vi "Contour Line_Find Intersected Edges.vi"(8 "height in":dbl, 9 "Z":dbl[][](array[numeric]), 10 "Y":dbl[][](array[numeric]), 11 "X":dbl[][](array[numeric])) -> (0 "height out":dbl, 2 "Intersected Edges":T1(array[cluster]), 3 "Contour Points":cluster{"x":dbl, "y":dbl}[](array[cluster]))   [LabVIEW 2020, in "NI_AAL_Geometry.lvlib"]
uses:
  <vilib>/Analysis/NI_AAL_Geometry.lvlib
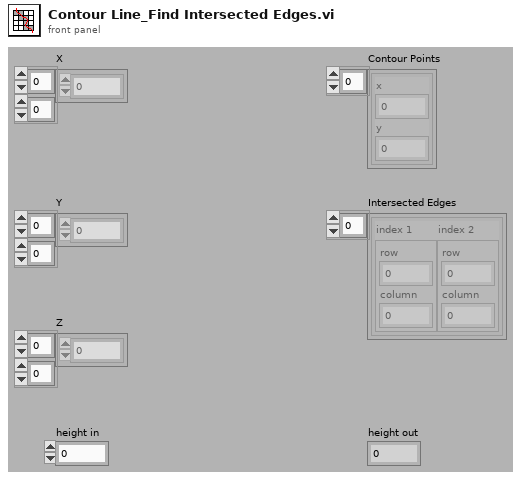
[diagram p1: front panel]
types:
  T1 = cluster{"index 1":cluster{"row":i32, "column":i32}, "index 2":cluster{"row":i32, "column":i32}}[]
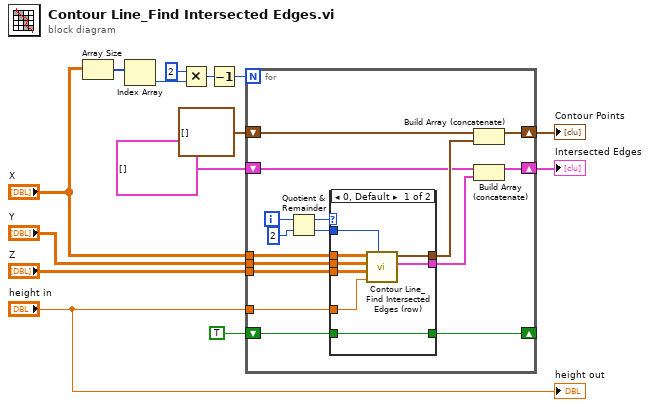
[diagram p0: block diagram]
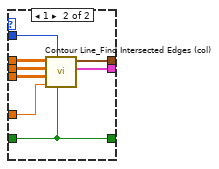
[diagram p2: hidden frame]
diagram:
  n1 = Array Size(array="X") -> (size(s)=w14:i32[])
  n2 = Index Array(array=w14) -> (element=w13:i32)  [unwired: 1 in]
  n3 = Multiply(x=2, y=w13) -> (x*y=w11:i32)
  n4 = Decrement(x=w11) -> (x-1=w10:i32)
  n5 = for {
    N: w10 -> [_]
    tunnel: "X" -> [w26]
    tunnel: "Y" -> [w25]
    tunnel: "height in" -> [w23]
    shift-right: [w20] -> w6
    shift-left: cluster{"x":dbl, "y":dbl}[] [] ("Contour Points 2") -> [w22]
    shift-right: [w17] -> w4
    shift-left: T1 [] ("Intersected Edges 2") -> [w19]
    shift-right: [w15] -> _
    shift-left: TRUE ("|/|? (F)") -> [w16]
    tunnel: "Z" -> [w24]
    i -> [w30]
    n6 = Quotient & Remainder(x=w30, y=2) -> (x-y*floor(x/y)=w28:i32, floor(x/y)=w27:i32)
    n7 = case shown="0, Default" w28 {
      tunnel: w27 -> [w34 w46]
      tunnel: w26 -> [w38 w45]
      tunnel: w25 -> [w37 w44]
      tunnel: w24 -> [w36 w43]
      tunnel: w23 -> [w35 w42]
      tunnel: [w33 w40] -> w21
      tunnel: [w32 w41] -> w18
      tunnel: w16 -> [w31 w39]
      tunnel: [w31 w39] -> w15
      frame 0, Default {
        n8 = call <vilib>:"Contour Line_Find Intersected Edges (row).vi"("row"=w34, "height"=w35, "Z"=w36, "Y"=w37, "X"=w38) -> ("Intersected Edges"=w32:T1, "Contour Points"=w33:cluster{"x":dbl, "y":dbl}[])  [unwired: 5 out]
      }
      frame 1 {
        n9 = call <vilib>:"Contour Line_Find Intersected Edges (col).vi"("|/|? (F)"=w39, "col"=w46, "height"=w42, "Z"=w43, "Y"=w44, "X"=w45) -> ("Intersected Edges"=w41:T1, "Contour Points"=w40:cluster{"x":dbl, "y":dbl}[])  [unwired: 4 out]
      }
    }
    n10 = Build Array (concatenate)(w22, w21) -> (w20:cluster{"x":dbl, "y":dbl}[])
    n11 = Build Array (concatenate)(w19, w18) -> (w17:T1)
  }
  "Intersected Edges" <- w4
  "Contour Points" <- w6
  "height out" <- "height in"
